vi "ATM Simulator.vi"() -> ()   [LabVIEW 2017]
doc: "This is a simulation of an Automated Teller Machine (ATM). It provides functionality for runtime-defined menus and functions, ATM card insertion and removal, and error handling."
uses:
  Controls/Buttons.ctl
  Controls/Menu.ctl
  Controls/ParcelLED.ctl
  Controls/UserInputState.ctl
  Controls/ConsumerControl.ctl
  Controls/ConsumerCommand.ctl
  Controls/DisplayControl.ctl
  Controls/DisplayCommand.ctl
  Controls/EnableDisableCommand.ctl
  Controls/UpdateMessageControl.ctl
  Controls/UpdateMessageCommand.ctl
  Controls/UpdateMenuCommand.ctl
  Controls/ElapsedTimeCommand.ctl
  Controls/MenuItem.ctl
  SubVIs/Global 2.vi
panel:
  out "UserInputState":T1
  out "Parcel number":string
  out "Phone number":string
  out "Cluster":T2
  in  "Right Buttons":T3
  out "Right Menu":T4
  out "Left Menu":T4
  out "ATM Messages":string
  in  "User Input":string
  in  "Enter":bool
  in  "Left Buttons":T3
  in  "Start Simulator":bool
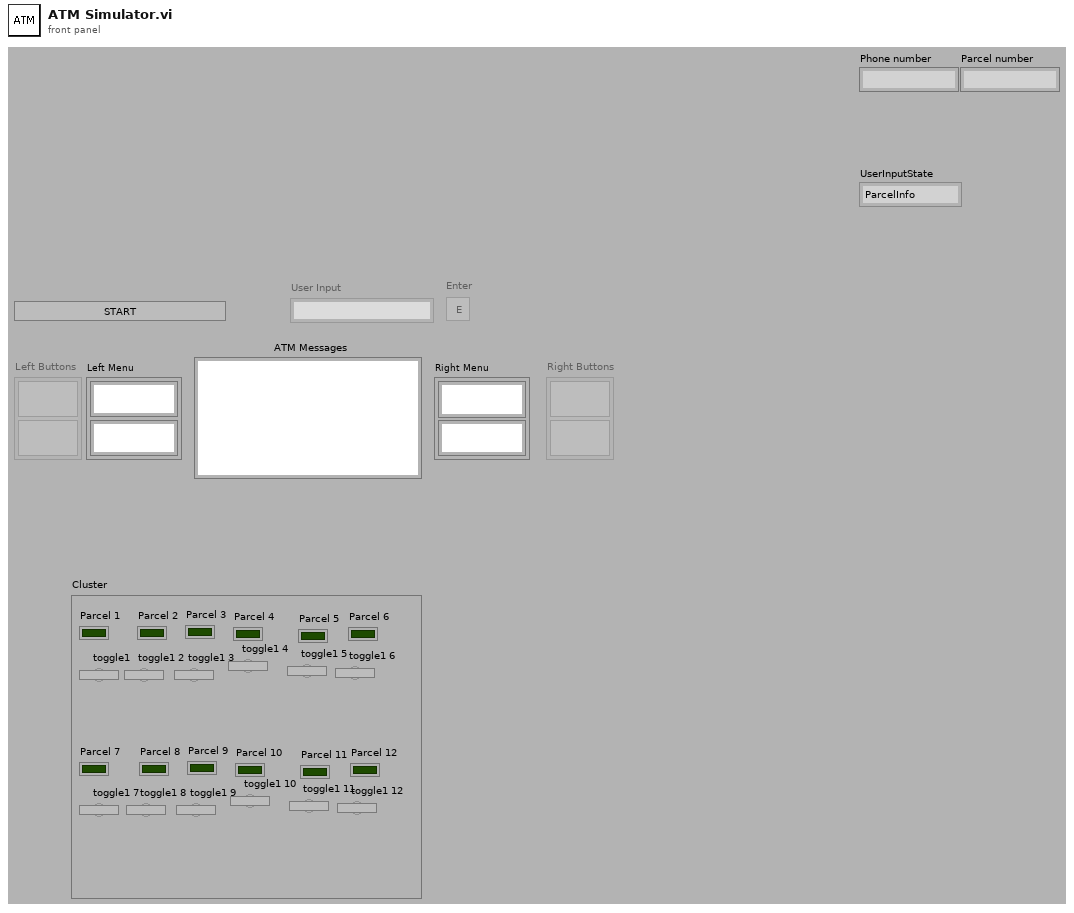
[diagram p1: front panel]
types:
  T1 = typedef "UserInputState.ctl" = enum16{"ParcelInfo", "PhoneInfo", "Deposit", "Withdrawal"}
  T2 = typedef "ParcelLED.ctl" = cluster{"Parcel 1":bool, "Parcel 2":bool, "Parcel 3":bool, "Parcel 4":bool, "Parcel 5":bool, "Parcel 6":bool, "Parcel 7":bool, "Parcel 8":bool, "Parcel 9":bool, "Parcel 10":bool, "Parcel 11":bool, "Parcel 12":bool, "toggle1":bool, "toggle1 2":bool, "toggle1 3":bool, "toggle1 4":bool, "toggle1 5":bool, "toggle1 6":bool, "toggle1 7":bool, "toggle1 8":bool, "toggle1 9":bool, "toggle1 10":bool, "toggle1 11":bool, "toggle1 12":bool}
  T3 = typedef "Buttons.ctl" = cluster{"Button 0":bool, "Button 1":bool}
  T4 = typedef "Menu.ctl" = cluster{"Menu 0":string, "Menu 1":string}
  T5 = typedef "DisplayControl.ctl" = cluster{"Command":T6, "Data":variant}
  T6 = typedef "DisplayCommand.ctl" = enum16{"Initialize", "Open/Close Parcel", "Enable/Disable Controls", "FocusCursor", "UpdateMessage", "UpdateMenus", "FinishOperation", "Exit", "CleanUserInput"}
  T7 = typedef "ConsumerControl.ctl" = cluster{"Command":T8, "Data":variant}
  T8 = typedef "ConsumerCommand.ctl" = enum16{"Initialize", "Start Operation", "User Input", "Left Button", "Right Button", "Exit"}
  T9 = typedef "ElapsedTimeCommand.ctl" = enum16{"Start", "CheckTime", "Stop"}
  T10 = typedef "MenuItem.ctl" = enum16{"Deposit", "Finish", "Withdraw", "None"}
  T11 = typedef "EnableDisableCommand.ctl" = enum16{"InitialSetup", "EnableUserInput", "DisableUserInput", "EnableMenus", "DisableMenus"}
  T12 = enum8{"Enabled", "Disabled", "Disabled and Grayed Out"}[]
  T13 = typedef "UpdateMessageControl.ctl" = cluster{"Command":T14, "Data":variant}
  T14 = typedef "UpdateMessageCommand.ctl" = enum16{"Welcome", "MainMenu", "PhoneNumberFailed", "PhoneNumberSuccess", "ParcelNumberSuccess", "ParcelNumbertFailed", "SessionTerminate", "SessionFinished", "Deposit", "DepositComplete", "Withdrawal", "WithdrawalComplete", "WithdrawalFailed"}
  T15 = typedef "Control 1.ctl" = string
  T16 = typedef "UpdateMenuCommand.ctl" = enum16{"MainMenu", "NoMenu"}
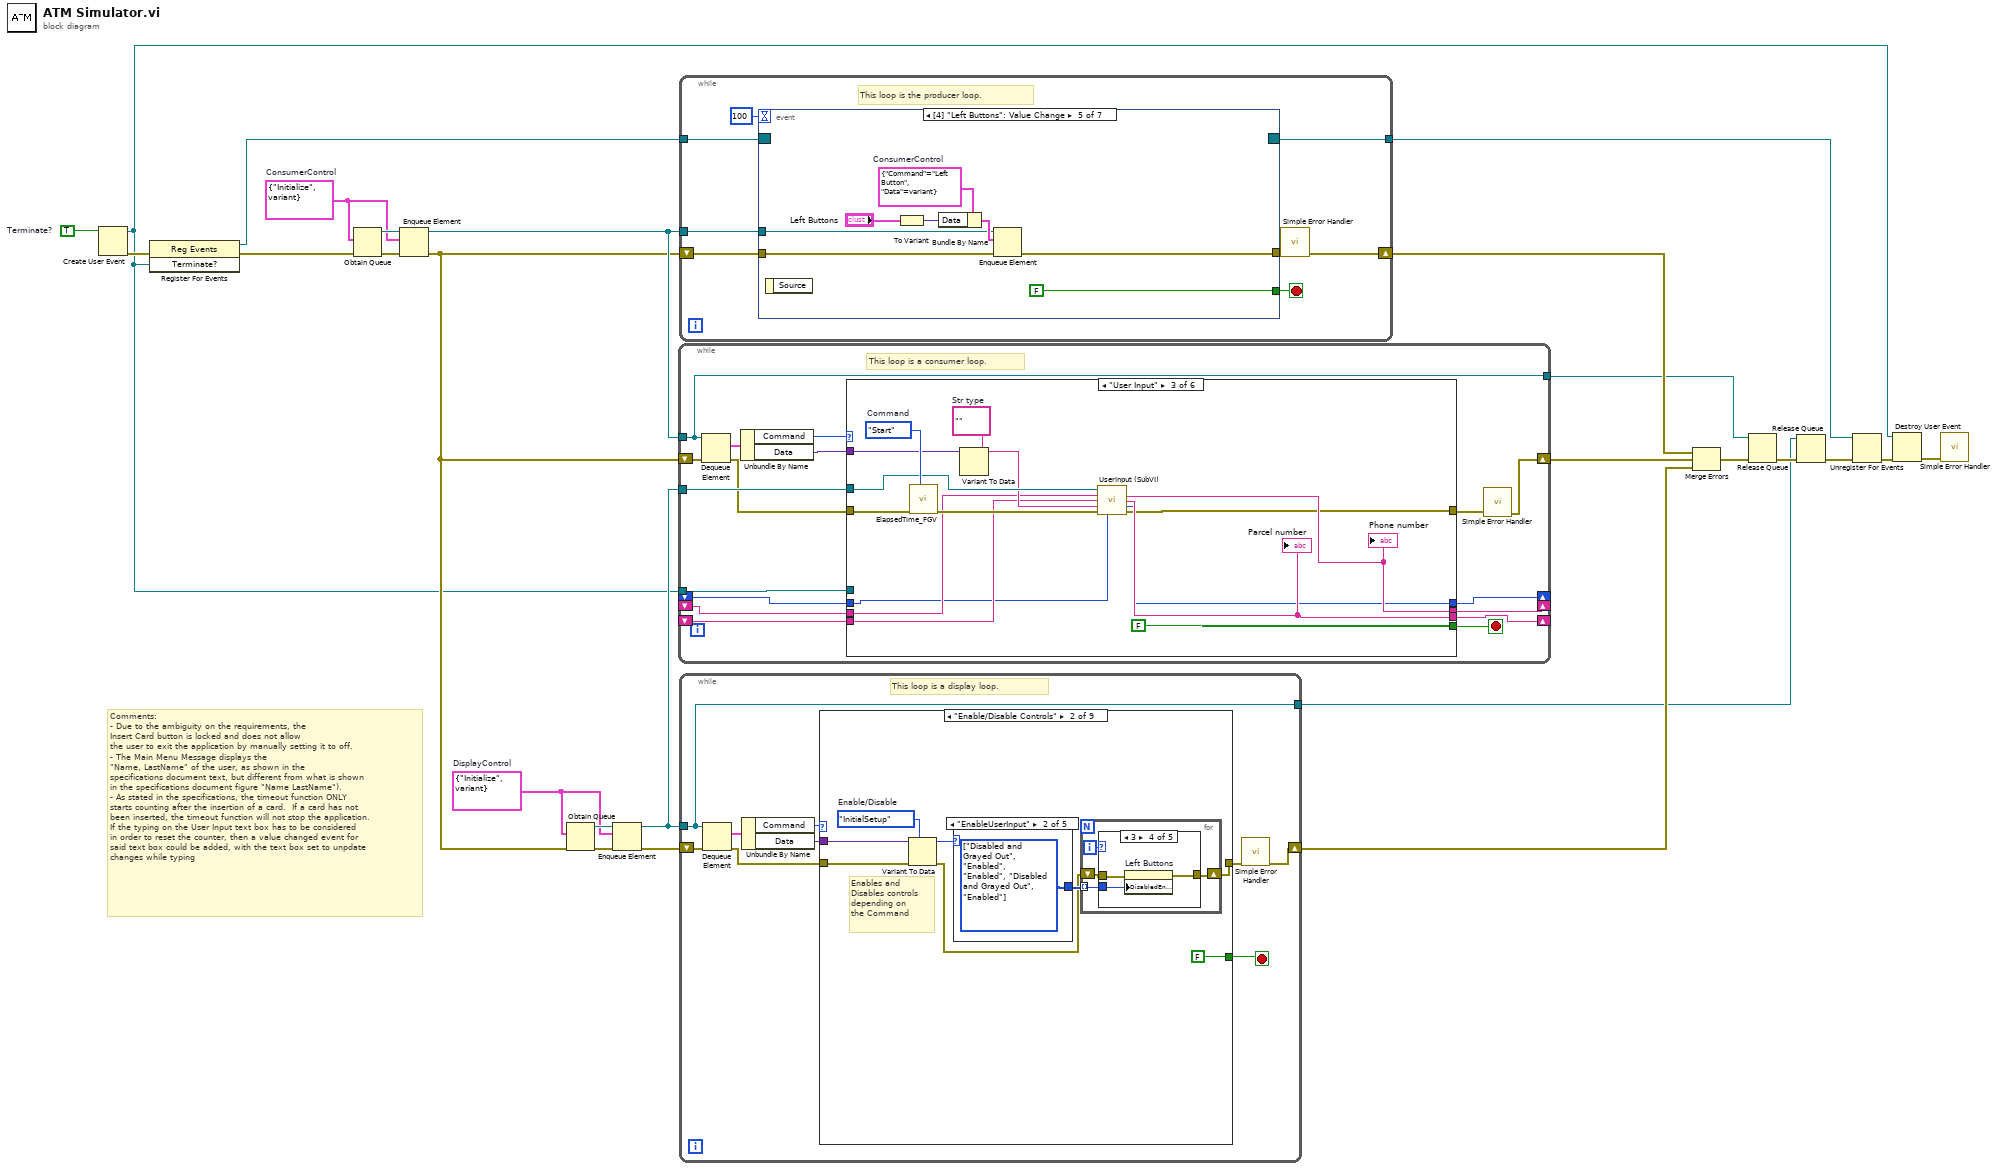
[diagram p0: block diagram]
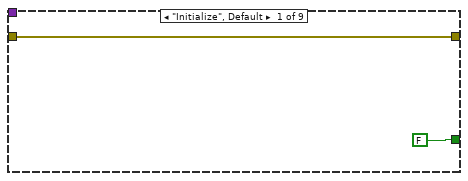
[diagram p2: hidden frame]
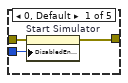
[diagram p3: hidden frame]
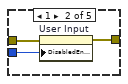
[diagram p4: hidden frame]
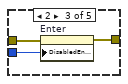
[diagram p5: hidden frame]
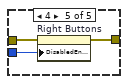
[diagram p6: hidden frame]
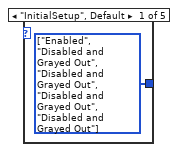
[diagram p7: hidden frame]
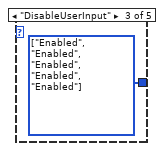
[diagram p8: hidden frame]
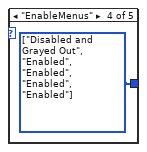
[diagram p9: hidden frame]
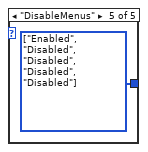
[diagram p10: hidden frame]
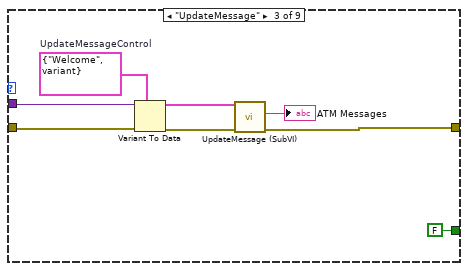
[diagram p11: hidden frame]
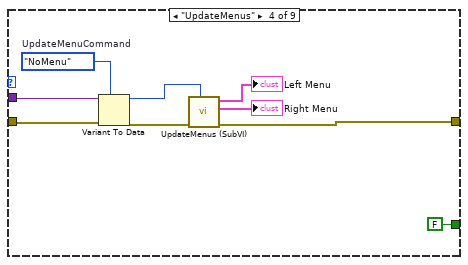
[diagram p12: hidden frame]
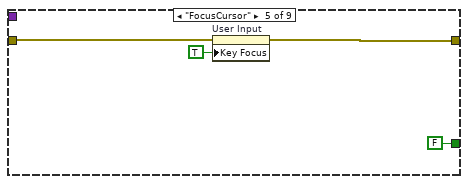
[diagram p13: hidden frame]
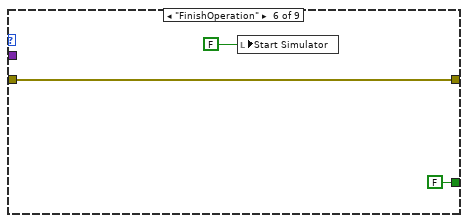
[diagram p14: hidden frame]
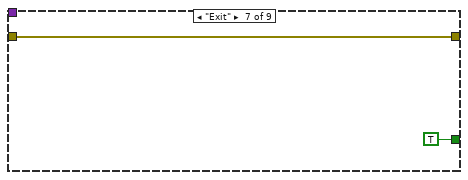
[diagram p15: hidden frame]
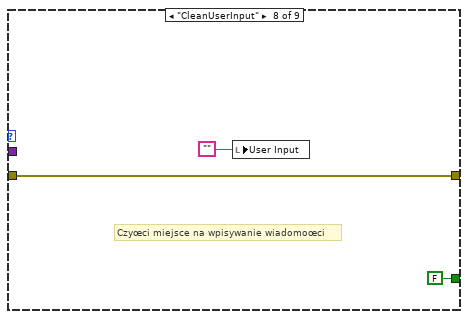
[diagram p16: hidden frame]
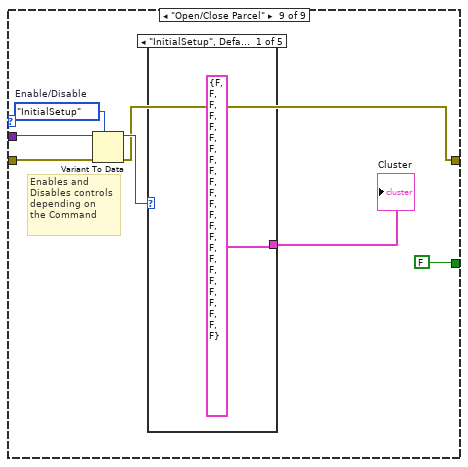
[diagram p17: hidden frame]
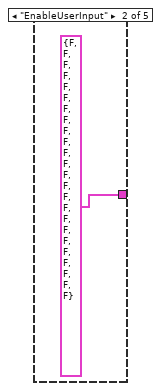
[diagram p18: hidden frame]
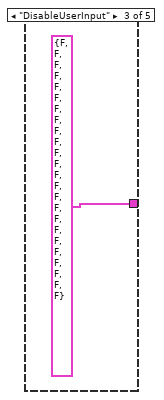
[diagram p19: hidden frame]
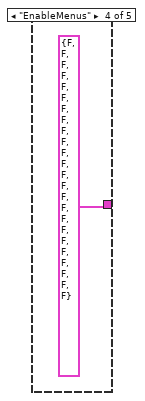
[diagram p20: hidden frame]
diagram:
  w9 = TRUE  # Terminate?
  w15 = T5 {"Command"=enum."Initialize", "Data"=variant}  # DisplayControl
  w23 = T7 {"Command"=enum."Initialize", "Data"=variant}  # ConsumerControl
  # "Comments:\n- Due to the ambiguity on the requirements, the\nInsert Card button is locked and does not allow\nthe user to exit the application by manually setting it to off.\n- The Main Menu Message displays the\n\"Name, LastName\" of the user, as shown in the\nspecifications document text, but different from what is shown \nin the specifications document figure \"Name LastName\").\n- As stated in the specifications, the timeout function ONLY\nstarts counting after the insertion of a card.  If a card has not\nbeen inserted, the timeout function will not stop the application.\nIf the typing on the User Input text box has to be considered\nin order to reset the counter, then a value changed event for\nsaid text box could be added, with the text box set to unpdate\nchanges while typing"
  n1 = Create User Event(user event datatype=w9) -> (user event=w1:refnum<user-event>, error out=w8:errorcluster)  [unwired: 1 in]
  n2 = register-events(error in=w8, w1) -> (reference out=w6:refnum<event-registration>, error out=w7:errorcluster)  [unwired: 1 in]
  n3 = Obtain Queue(element data type=w23, error in (no error)=w7) -> (queue out=w26:refnum<queue>, error out=w25:errorcluster)  [unwired: 3 in, 1 out]
  n4 = Enqueue Element(queue=w26, element=w23, error in (no error)=w25) -> (queue out=w24:refnum<queue>, error out=w2:errorcluster)  [unwired: 1 in, 1 out]
  n5 = Obtain Queue(element data type=w15, error in (no error)=w2) -> (queue out=w16:refnum<queue>, error out=w17:errorcluster)  [unwired: 3 in, 1 out]
  n6 = Enqueue Element(queue=w16, element=w15, error in (no error)=w17) -> (queue out=w11:refnum<queue>, error out=w14:errorcluster)  [unwired: 1 in, 1 out]
  n7 = while {
    tunnel: w24 -> [w40]
    tunnel: [w40] -> w19
    shift-right: [w30] -> w18
    shift-left: w2 -> [w39]
    tunnel: w11 -> [w38]
    shift-right: [w34] -> _
    shift-left: _ -> [w35]
    shift-right: [w32] -> _
    shift-left: _ -> [w33]
    tunnel: w1 -> [w31]
    shift-right: [w28] -> _
    shift-left: _ -> [w27]
    stop <- w41 stop-if-true
    # "This loop is a consumer loop."
    n8 = Dequeue Element(queue=w40, error in (no error)=w39) -> (element=w43:T7, error out=w36:errorcluster)  [unwired: 1 in, 2 out]
    n9 = Unbundle By Name(w43) -> ("Command"=w42:T8, "Data"=w37:variant)
    n10 = case shown="\"User Input\"" w42 {
      tunnel: [FALSE FALSE FALSE FALSE FALSE TRUE] -> w41
      tunnel: w38 -> [w49 w59 w66 w90 w108 w121]
      tunnel: w37 -> [_ _ w71 w89 w107 _]
      tunnel: w36 -> [w50 w58 w74 w93 w112 w120]
      tunnel: w35 -> [w46 _ w61 w82 w98 w117]
      tunnel: [w46 UserInputState."PhoneInfo" ("UserInputState") w60 w75 w109 w117] -> w34
      tunnel: w33 -> [w47 w56 w62 w81 w97 w119]
      tunnel: [w47 w56 w69 w81 w97 w119] -> w32
      tunnel: w31 -> [_ _ _ w80 w96 _]
      tunnel: [w45 w52 w67 w78 w95 w114] -> w29
      tunnel: [w44 w51 w68 w77 w94 w113] -> w28
      tunnel: w27 -> [w44 w51 w63 w77 w94 w113]
      frame "Initialize", Default {
        n11 = call "InitializeDisplay (SubVI).vi"("error in (no error)"=w50, "Display Queue in"=w49) -> ("error out"=w45:errorcluster)  [unwired: 8 in, 1 out]
      }
      frame "Start Operation" {
        w57 = ElapsedTimeCommand."Start"  # UserInputState
        n12 = call "StartOperation (SubVI).vi"("error in (no error)"=w58, "Display Queue in"=w59) -> ("error out"=w54:errorcluster)  [unwired: 8 in, 1 out]
        n13 = call "ElapsedTime_FGV.vi"("Command"=w57, "Error In"=w54) -> ("Error Out"=w52:errorcluster)  [unwired: 7 in, 2 out]
      }
      frame "User Input" {
        w72 = ""  # Str type
        w73 = ElapsedTimeCommand."Start"  # Command
        n14 = call "ElapsedTime_FGV.vi"("Command"=w73, "Error In"=w74) -> ("Error Out"=w64:errorcluster)  [unwired: 7 in, 2 out]
        n15 = Variant To Data(type=w72, Variant=w71) -> (data=w65:string)  [unwired: 1 in, 1 out]
        n16 = call "UserInput (SubVI).vi"("Display Queue In"=w66, "Phone number"=w62, "Parcel number"=w63, "User Input"=w65, "Error In"=w64, "UserInputState"=w61) -> ("Phone number"=w69:string, "Parcel number"=w68:string, "UserInputState 3"=w60:T1, "Error Out"=w67:errorcluster)  [unwired: 5 in, 1 out]
        "Phone number" <- w69
        "Parcel number" <- w68
      }
      frame "Left Button" {
        w79 = T10[] [enum."Withdraw", enum."Deposit", enum."Withdraw"] items=["Deposit", "Finish", "Withdraw", "None"]  # MenuItemsArray
        w87 = T3 {"Button 0"=FALSE, "Button 1"=FALSE}  # Left Buttons
        w92 = ElapsedTimeCommand."Start"  # Command
        n17 = call "ElapsedTime_FGV.vi"("Command"=w92, "Error In"=w93) -> ("Error Out"=w83:errorcluster)  [unwired: 7 in, 2 out]
        n18 = Variant To Data(type=w87, Variant=w89) -> (data=w88:T3)  [unwired: 1 in, 1 out]
        n19 = Cluster To Array(cluster=w88) -> (array=w86:bool[])
        n20 = Search 1D Array(1D array=w86, element=TRUE) -> (index of element=w84:i32)  [unwired: 1 in]
        n21 = Index Array(array=w79, index=w84) -> (element=w76:T10)
        n22 = call "MenuItem (SubVI).vi"("UserEvent In"=w80, "MenuItem"=w76, "error in (no error)"=w83, "Account"=w81, "UserInputState"=w82, "Display Queue in"=w90) -> ("error out"=w78:errorcluster, "UserInputState"=w75:T1)  [unwired: 3 in, 1 out]
        "UserInputState" <- w75
        n23 = global write "Global 2.vi" "element"(w76) -> ()
      }
      frame "Right Button" {
        w99 = T3 {"Button 0"=FALSE, "Button 1"=FALSE}  # Right Buttons
        w102 = T10[] [enum."None", enum."Finish", enum."Withdraw"] items=["Deposit", "Finish", "Withdraw", "None"]  # MenuItemsArray
        w111 = ElapsedTimeCommand."Start"  # Command
        n24 = call "ElapsedTime_FGV.vi"("Command"=w111, "Error In"=w112) -> ("Error Out"=w100:errorcluster)  [unwired: 7 in, 2 out]
        n25 = Variant To Data(type=w99, Variant=w107) -> (data=w106:T3)  [unwired: 1 in, 1 out]
        n26 = Cluster To Array(cluster=w106) -> (array=w105:bool[])
        n27 = Search 1D Array(1D array=w105, element=TRUE) -> (index of element=w103:i32)  [unwired: 1 in]
        n28 = Index Array(array=w102, index=w103) -> (element=w101:T10)
        n29 = call "MenuItem (SubVI).vi"("UserEvent In"=w96, "MenuItem"=w101, "error in (no error)"=w100, "Account"=w97, "UserInputState"=w98, "Display Queue in"=w108) -> ("error out"=w95:errorcluster, "UserInputState"=w109:T1)  [unwired: 3 in, 1 out]
      }
      frame "Exit" {
        w115 = ElapsedTimeCommand."Stop"  # Command
        n30 = call "ExitApp (SubVI).vi"("error in (no error)"=w120, "Display Queue in"=w121) -> ("error out"=w116:errorcluster)  [unwired: 8 in, 1 out]
        n31 = call "ElapsedTime_FGV.vi"("Command"=w115, "Error In"=w116) -> ("Error Out"=w114:errorcluster)  [unwired: 7 in, 2 out]
      }
    }
    n32 = call <vilib>:"Simple Error Handler.vi"("error in (no error)"=w29) -> ("error out"=w30:errorcluster)  [unwired: 4 in, 4 out]
  }
  n33 = while {
    shift-right: [w124] -> w20
    shift-left: w2 -> [w128]
    tunnel: w24 -> [w129]
    tunnel: w6 -> [w123]
    tunnel: [w122] -> w4
    stop <- w127 stop-if-true
    # "This loop is the producer loop."
    n34 = event shown="[4] \"Left Buttons\": Value Change" {
      selector: w123 -> [_ _ _ _ _ _ _]
      dyn-events: [_ _ _ _ _ _ _] -> w122
      timeout: 100 -> [_ _ _ _ _ _ _]
      tunnel: w129 -> [w133 w146 w153 w165 w169 w177 w184]
      tunnel: w128 -> [w137 w147 w152 w166 w170 w178 w185]
      tunnel: [w134 w145 w150 w159 w171 w179 w183] -> w125
      tunnel: [w132 _ FALSE ("stop") FALSE ("stop") FALSE ("stop") FALSE ("stop") TRUE ("stop")] -> w127
      event Timeout {
        w136 = u32 10  # DesiredTime (s)
        w131 = ElapsedTimeCommand."CheckTime"  # Command
        # "Stop only is\nthe timer has expired"
        n35 = event-data() -> ()  [unwired: 1 in, 1 out]
        n36 = call "ElapsedTime_FGV.vi"("Command"=w131, "Error In"=w137, "DesiredTime (s)"=w136) -> ("Error Out"=w135:errorcluster, "Done?"=w130:bool)  [unwired: 6 in, 1 out]
        n37 = case shown="True" w130 {
          tunnel: w135 -> [w139 w144]
          tunnel: [w139 w143] -> w134
          tunnel: w133 -> [_ w142]
          tunnel: [FALSE ("stop") TRUE ("stop")] -> w132
          frame False {
          }
          frame True {
            w141 = T7 {"Command"=enum."Exit", "Data"=variant}  # ConsumerControl
            n38 = Enqueue Element(queue=w142, element=w141, error in (no error)=w144) -> (error out=w143:errorcluster)  [unwired: 1 in, 2 out]
          }
        }
      }
      event Value Change {
        w148 = T7 {"Command"=enum."Exit", "Data"=variant}  # ConsumerControl
        n39 = event-data() -> ()  [unwired: 1 in, 1 out]
        n40 = Enqueue Element(queue=w146, element=w148, error in (no error)=w147) -> (error out=w145:errorcluster)  [unwired: 1 in, 2 out]
      }
      event "Start Simulator": Value Change {
        n41 = event-data() -> ()  [unwired: 1 in, 1 out]
        n42 = case shown="True" "Start Simulator" {
          tunnel: w153 -> [_ w158]
          tunnel: w152 -> [w154 w157]
          tunnel: [w154 w155] -> w150
          frame False {
          }
          frame True {
            w156 = T7 {"Command"=enum."Start Operation", "Data"=variant}  # ConsumerControl
            n43 = Enqueue Element(queue=w158, element=w156, error in (no error)=w157) -> (error out=w155:errorcluster)  [unwired: 1 in, 2 out]
          }
        }
      }
      event "Enter": Value Change {
        w164 = T7 {"Command"=enum."User Input", "Data"=variant}  # ConsumerControl
        n44 = event-data() -> ()  [unwired: 1 in, 1 out]
        n45 = To Variant(anything="User Input") -> (Variant=w162:variant)
        n46 = Bundle By Name(cluster=w164, "Data"=w162) -> (w163:T7)
        n47 = Enqueue Element(queue=w165, element=w163, error in (no error)=w166) -> (error out=w159:errorcluster)  [unwired: 1 in, 2 out]
      }
      event Value Change {
        w174 = T7 {"Command"=enum."Left Button", "Data"=variant}  # ConsumerControl
        n48 = event-data() -> ()  [unwired: 1 in, 1 out]
        n49 = To Variant(anything="Left Buttons") -> (Variant=w172:variant)
        n50 = Bundle By Name(cluster=w174, "Data"=w172) -> (w173:T7)
        n51 = Enqueue Element(queue=w169, element=w173, error in (no error)=w170) -> (error out=w171:errorcluster)  [unwired: 1 in, 2 out]
      }
      event Value Change {
        w182 = T7 {"Command"=enum."Right Button", "Data"=variant}  # ConsumerControl
        n52 = event-data() -> ()  [unwired: 1 in, 1 out]
        n53 = To Variant(anything="Right Buttons") -> (Variant=w180:variant)
        n54 = Bundle By Name(cluster=w182, "Data"=w180) -> (w181:T7)
        n55 = Enqueue Element(queue=w177, element=w181, error in (no error)=w178) -> (error out=w179:errorcluster)  [unwired: 1 in, 2 out]
      }
      event User Event {
        w186 = T7 {"Command"=enum."Exit", "Data"=variant}  # ConsumerControl
        n56 = event-data() -> ()  [unwired: 1 in, 1 out]
        n57 = Enqueue Element(queue=w184, element=w186, error in (no error)=w185) -> (error out=w183:errorcluster)  [unwired: 1 in, 2 out]
      }
    }
    n58 = call <vilib>:"Simple Error Handler.vi"("error in (no error)"=w125) -> ("error out"=w124:errorcluster)  [unwired: 4 in, 4 out]
  }
  n59 = while {
    tunnel: w11 -> [w194]
    tunnel: [w194] -> w12
    shift-right: [w193] -> w13
    shift-left: w14 -> [w192]
    stop <- w189 stop-if-true
    # "This loop is a display loop."
    n60 = Dequeue Element(queue=w194, error in (no error)=w192) -> (element=w196:T5, error out=w190:errorcluster)  [unwired: 1 in, 2 out]
    n61 = Unbundle By Name(w196) -> ("Command"=w195:T6, "Data"=w191:variant)
    n62 = case shown="\"Enable/Disable Controls\"" w195 {
      tunnel: [FALSE FALSE FALSE FALSE FALSE FALSE TRUE FALSE FALSE] -> w189
      tunnel: w191 -> [_ w206 w238 w246 _ _ _ _ w262]
      tunnel: w190 -> [w197 w204 w237 w247 w251 w252 w255 w258 w263]
      tunnel: [w197 w199 w232 w240 w250 w252 w255 w258 w261] -> w188
      frame "Initialize", Default {
      }
      frame "Enable/Disable Controls" {
        w205 = EnableDisableCommand."InitialSetup"  # Enable/Disable
        # "Enables and\nDisables controls\ndepending on\nthe Command"
        n63 = Variant To Data(error in=w204, type=w205, Variant=w206) -> (data=w203:T11, error out=w200:errorcluster)
        n64 = case shown="\"EnableUserInput\"" w203 {
          tunnel: [w226 w227 w228 w229 w230] -> w201
          frame "InitialSetup", Default {
            w226 = T12 [enum."Enabled", enum."Disabled and Grayed Out", enum."Disabled and Grayed Out", enum."Disabled and Grayed Out", enum."Disabled and Grayed Out"] items=["Enabled", "Disabled", "Disabled and Grayed Out"]
          }
          frame "EnableUserInput" {
            w227 = T12 [enum."Disabled and Grayed Out", enum."Enabled", enum."Enabled", enum."Disabled and Grayed Out", enum."Enabled"] items=["Enabled", "Disabled", "Disabled and Grayed Out"]
          }
          frame "DisableUserInput" {
            w228 = T12 [enum."Enabled", enum."Enabled", enum."Enabled", enum."Enabled", enum."Enabled"] items=["Enabled", "Disabled", "Disabled and Grayed Out"]
          }
          frame "EnableMenus" {
            w229 = T12 [enum."Disabled and Grayed Out", enum."Enabled", enum."Enabled", enum."Enabled", enum."Enabled"] items=["Enabled", "Disabled", "Disabled and Grayed Out"]
          }
          frame "DisableMenus" {
            w230 = T12 [enum."Enabled", enum."Disabled", enum."Disabled", enum."Disabled", enum."Disabled"] items=["Enabled", "Disabled", "Disabled and Grayed Out"]
          }
        }
        n65 = for {
          tunnel: w201 -> [w209] mode=indexing
          shift-right: [w207] -> w199
          shift-left: w200 -> [w208]
          i -> [w210]
          n66 = case shown="3" w210 {
            tunnel: w209 -> [w213 w216 w219 w222 w225]
            tunnel: w208 -> [w212 w215 w218 w221 w224]
            tunnel: [w211 w214 w217 w220 w223] -> w207
            frame 0, Default {
              n67 = property on="Start Simulator" class="Bool (strict)"(error in=w212, "DisabledEnum"=w213) -> (error out=w211:errorcluster)  [unwired: 1 in, 1 out]
            }
            frame 1 {
              n68 = property on="User Input" class="Str"(error in=w215, "DisabledEnum"=w216) -> (error out=w214:errorcluster)  [unwired: 1 in, 1 out]
            }
            frame 2 {
              n69 = property on="Enter" class="Bool"(error in=w218, "DisabledEnum"=w219) -> (error out=w217:errorcluster)  [unwired: 1 in, 1 out]
            }
            frame 3 {
              n70 = property on="Left Buttons" class="Clust"(error in=w221, "DisabledEnum"=w222) -> (error out=w220:errorcluster)  [unwired: 1 in, 1 out]
            }
            frame 4 {
              n71 = property on="Right Buttons" class="Clust"(error in=w224, "DisabledEnum"=w225) -> (error out=w223:errorcluster)  [unwired: 1 in, 1 out]
            }
          }
        }
      }
      frame "UpdateMessage" {
        w236 = T13 {"Command"=enum."Welcome", "Data"=variant}  # UpdateMessageControl
        n72 = Variant To Data(error in=w237, type=w236, Variant=w238) -> (data=w235:T13, error out=w233:errorcluster)
        n73 = call "UpdateMessage (SubVI).vi"("Error In"=w233, "UpdateMessageControl"=w235) -> ("Error Out"=w232:errorcluster, "ATM Messages"=→"ATM Messages":T15)  [unwired: 8 in]
      }
      frame "UpdateMenus" {
        w245 = UpdateMenuCommand."NoMenu"  # UpdateMenuCommand
        n74 = Variant To Data(error in=w247, type=w245, Variant=w246) -> (data=w244:T16, error out=w243:errorcluster)
        n75 = call "UpdateMenus (SubVI).vi"("UpdateMenuCommand"=w244, "Error In"=w243) -> ("Error Out"=w240:errorcluster, "Right Menu"=→"Right Menu":T4, "Left Menu"=→"Left Menu":T4)  [unwired: 7 in]
      }
      frame "FocusCursor" {
        n76 = property on="User Input" class="Str"(error in=w251, "Key Focus"=TRUE) -> (error out=w250:errorcluster)  [unwired: 1 in, 1 out]
      }
      frame "FinishOperation" {
        n77 = local write "Start Simulator"(FALSE ("Card Simulator")) -> ()
      }
      frame "Exit" {
      }
      frame "CleanUserInput" {
        # "Czyœci miejsce na wpisywanie wiadomoœci"
        n78 = local write "User Input"("") -> ()
      }
      frame "Open/Close Parcel" {
        w266 = EnableDisableCommand."InitialSetup"  # Enable/Disable
        # "Enables and\nDisables controls\ndepending on\nthe Command"
        n79 = Variant To Data(error in=w263, type=w266, Variant=w262) -> (data=w265:T11, error out=w261:errorcluster)
        n80 = case shown="\"InitialSetup\", Default" w265 {
          tunnel: [T2 {"Parcel 1"=FALSE, "Parcel 2"=FALSE, "Parcel 3"=FALSE, "Parcel 4"=FALSE, "Parcel 5"=FALSE, "Parcel 6"=FALSE, "Parcel 7"=FALSE, "Parcel 8"=FALSE, "Parcel 9"=FALSE, "Parcel 10"=FALSE, "Parcel 11"=FALSE, "Parcel 12"=FALSE, "toggle1"=FALSE, "toggle1 2"=FALSE, "toggle1 3"=FALSE, "toggle1 4"=FALSE, "toggle1 5"=FALSE, "toggle1 6"=FALSE, "toggle1 7"=FALSE, "toggle1 8"=FALSE, "toggle1 9"=FALSE, "toggle1 10"=FALSE, "toggle1 11"=FALSE, "toggle1 12"=FALSE} ("Cluster") T2 {"Parcel 1"=FALSE, "Parcel 2"=FALSE, "Parcel 3"=FALSE, "Parcel 4"=FALSE, "Parcel 5"=FALSE, "Parcel 6"=FALSE, "Parcel 7"=FALSE, "Parcel 8"=FALSE, "Parcel 9"=FALSE, "Parcel 10"=FALSE, "Parcel 11"=FALSE, "Parcel 12"=FALSE, "toggle1"=FALSE, "toggle1 2"=FALSE, "toggle1 3"=FALSE, "toggle1 4"=FALSE, "toggle1 5"=FALSE, "toggle1 6"=FALSE, "toggle1 7"=FALSE, "toggle1 8"=FALSE, "toggle1 9"=FALSE, "toggle1 10"=FALSE, "toggle1 11"=FALSE, "toggle1 12"=FALSE} ("Cluster") T2 {"Parcel 1"=FALSE, "Parcel 2"=FALSE, "Parcel 3"=FALSE, "Parcel 4"=FALSE, "Parcel 5"=FALSE, "Parcel 6"=FALSE, "Parcel 7"=FALSE, "Parcel 8"=FALSE, "Parcel 9"=FALSE, "Parcel 10"=FALSE, "Parcel 11"=FALSE, "Parcel 12"=FALSE, "toggle1"=FALSE, "toggle1 2"=FALSE, "toggle1 3"=FALSE, "toggle1 4"=FALSE, "toggle1 5"=FALSE, "toggle1 6"=FALSE, "toggle1 7"=FALSE, "toggle1 8"=FALSE, "toggle1 9"=FALSE, "toggle1 10"=FALSE, "toggle1 11"=FALSE, "toggle1 12"=FALSE} ("Cluster") T2 {"Parcel 1"=FALSE, "Parcel 2"=FALSE, "Parcel 3"=FALSE, "Parcel 4"=FALSE, "Parcel 5"=FALSE, "Parcel 6"=FALSE, "Parcel 7"=FALSE, "Parcel 8"=FALSE, "Parcel 9"=FALSE, "Parcel 10"=FALSE, "Parcel 11"=FALSE, "Parcel 12"=FALSE, "toggle1"=FALSE, "toggle1 2"=FALSE, "toggle1 3"=FALSE, "toggle1 4"=FALSE, "toggle1 5"=FALSE, "toggle1 6"=FALSE, "toggle1 7"=FALSE, "toggle1 8"=FALSE, "toggle1 9"=FALSE, "toggle1 10"=FALSE, "toggle1 11"=FALSE, "toggle1 12"=FALSE} ("Cluster") T2 {"Parcel 1"=FALSE, "Parcel 2"=FALSE, "Parcel 3"=FALSE, "Parcel 4"=FALSE, "Parcel 5"=FALSE, "Parcel 6"=FALSE, "Parcel 7"=FALSE, "Parcel 8"=FALSE, "Parcel 9"=FALSE, "Parcel 10"=FALSE, "Parcel 11"=FALSE, "Parcel 12"=FALSE, "toggle1"=FALSE, "toggle1 2"=FALSE, "toggle1 3"=FALSE, "toggle1 4"=FALSE, "toggle1 5"=FALSE, "toggle1 6"=FALSE, "toggle1 7"=FALSE, "toggle1 8"=FALSE, "toggle1 9"=FALSE, "toggle1 10"=FALSE, "toggle1 11"=FALSE, "toggle1 12"=FALSE} ("Cluster")] -> w260
          frame "InitialSetup", Default {
          }
          frame "EnableUserInput" {
          }
          frame "DisableUserInput" {
          }
          frame "EnableMenus" {
          }
          frame "DisableMenus" {
          }
        }
        "Cluster" <- w260
      }
    }
    n81 = call <vilib>:"Simple Error Handler.vi"("error in (no error)"=w188) -> ("error out"=w193:errorcluster)  [unwired: 4 in, 4 out]
  }
  n82 = Merge Errors(w20, w18, w13) -> (w21:errorcluster)
  n83 = Release Queue(queue=w19, error in (no error)=w21) -> (error out=w22:errorcluster)  [unwired: 1 in, 2 out]
  n84 = Release Queue(queue=w12, error in (no error)=w22) -> (error out=w5:errorcluster)  [unwired: 1 in, 2 out]
  n85 = Unregister For Events(event registration refnum=w4, error in=w5) -> (error out=w10:errorcluster)
  n86 = Destroy User Event(user event=w1, error in=w10) -> (error out=w3:errorcluster)
  n87 = call <vilib>:"Simple Error Handler.vi"("error in (no error)"=w3) -> ()  [unwired: 4 in, 5 out]
